vi "Hardware - TDK Lambda HV PS Control.vi"() -> ()   [LabVIEW 2015, in "ECS-Host.lvlib"]
uses:
  ECS-Host.lvlib
panel:
  in  "GEN Control Loop Rate Set":u32 caption="[]"
  out "GEN Control Loop Duration":sgl caption="[V]" format="%#.2g"
  out "OverVoltage Limit":sgl caption="[V]" format="%#.2g"
  out "GEN Error Source":string
  out "GEN Error Code":i32
  out "GEN Error Status":bool
  out "_TDK Error":T1 caption="TDK Error"
  out "GEN Control Mode":enum32{"LOCAL", "REMOTE", "LOCKOUT"}(ring)
  in  "Reset":bool
  in  "GEN Address":i32 caption="[]"
  in  "GEN BaudRate":enum32{"1200", "2400", "4800", "9600", "19200"}(ring)
  out "GEN Current Output":sgl caption="[A]" format="%#.2g"
  out "GEN Voltage Output":sgl caption="[]" format="%#.2g"
  in  "Output Enable":bool
  in  "GEN Current Limit":sgl caption="[A]" format="%#.2g"
  in  "GEN Voltage Setpoint":sgl caption="[]" format="%#.2g"
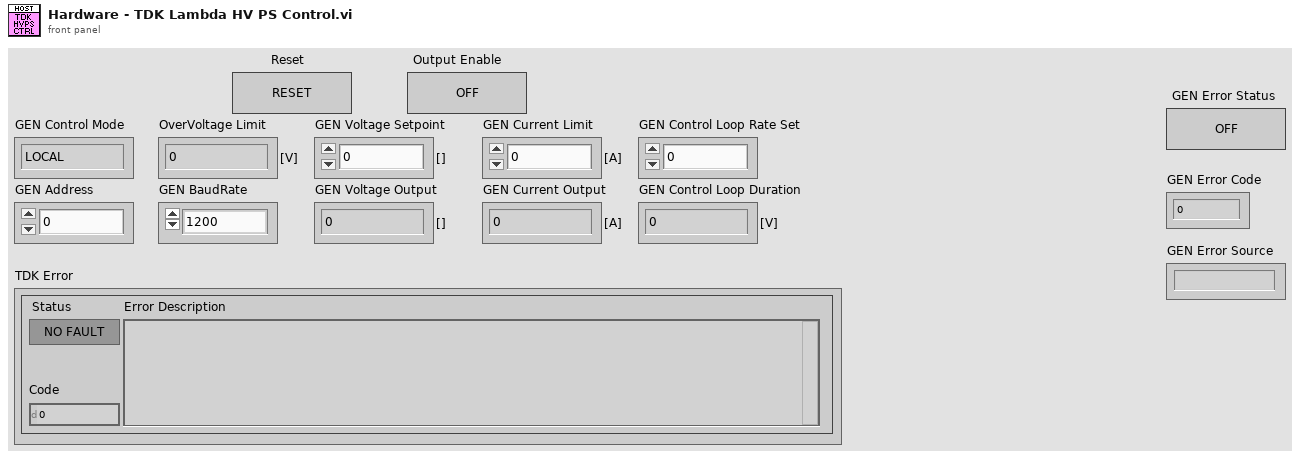
[diagram p1: front panel]
types:
  T1 = cluster{"Status":bool, "Code":i32, "Error Description":string}
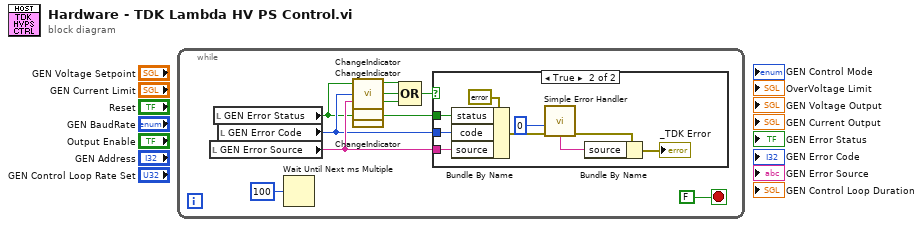
[diagram p0: block diagram]
diagram:
  n1 = while {
    stop <- FALSE stop-if-true
    n2 = local read "GEN Error Source"() -> (w4:string)
    n3 = local read "GEN Error Status"() -> (w2:bool)
    n4 = local read "GEN Error Code"() -> (w3:i32)
    n5 = Wait Until Next ms Multiple(millisecond multiple=u32 100) -> ()  [unwired: 1 out]
    n6 = call "ChangeIndicator.vi"("Input"=w2) -> ("Change"=w5:bool)  [unwired: 9 in]
    n7 = call "ChangeIndicator.vi"("Input"=w3) -> ("Change"=w6:bool)  [unwired: 9 in]
    n8 = call "ChangeIndicator.vi"("Input"=w4) -> ("Change"=w7:bool)  [unwired: 9 in]
    n9 = Compound Arithmetic op=OR(w5, w6, w7) -> (w8:bool)
    n10 = case shown="True" w8 {
      tunnel: w2 -> [_ w18]
      tunnel: w3 -> [_ w17]
      tunnel: w4 -> [_ w16]
      frame False {
      }
      frame True {
        n11 = Bundle By Name(cluster=errorcluster {"status"=FALSE, "code"=0, "source"=""} ("error out"), "status"=w18, "code"=w17, "source"=w16) -> (w15:errorcluster)
        n12 = call <vilib>:"Simple Error Handler.vi"("type of dialog (OK msg:1)"=i16 0, "error in (no error)"=w15) -> ("error out"=w12:errorcluster, "message"=w13:string)  [unwired: 3 in, 3 out]
        n13 = Bundle By Name(cluster=w12, "source"=w13) -> (→"_TDK Error":errorcluster)
      }
    }
  }
